vi "Read Images.vi"(8 "error in":errorcluster, 11 "Communicator Worker in":refnum<class "Camera Worker.lvclass">) -> (0 "error out":errorcluster, 3 "Communicator Worker out":refnum<class "Camera Worker.lvclass">)   [LabVIEW 2020, in "Camera Worker.lvlib" / "Camera Worker.lvclass"]
doc: "This method copies images from the camera's driver buffer into a local one."
uses:
  Camera Worker.lvclass
  Camera Worker.lvclass/Camera Worker.ctl
  Interfaces/IRead Image/IRead Images/IRead Image.lvclass
panel:
  out "Exec Time (ms)":u32
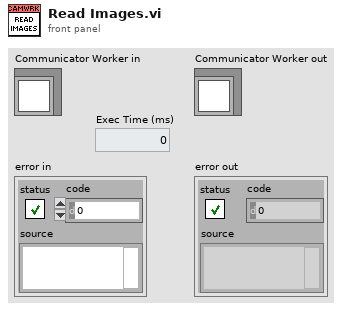
[diagram p1: front panel]
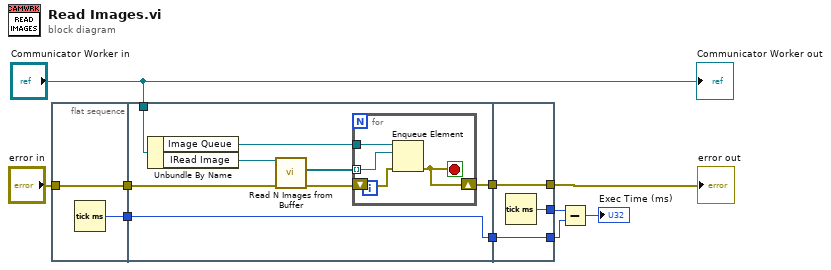
[diagram p0: block diagram]
diagram:
  n1 = flat-sequence {
    tunnel: "error in" -> [w12]
    tunnel: [w12] -> w7
    tunnel: [w11] -> w3
    tunnel: "Communicator Worker in" -> [w20]
    tunnel: w7 -> [w19]
    tunnel: [w16] -> w6
    tunnel: w3 -> [w13]
    tunnel: [w13] -> w2
    tunnel: [w27] -> w8
    tunnel: w6 -> [w27]
    tunnel: [w26] -> w5
    tunnel: [w25] -> w4
    tunnel: w2 -> [w25]
    frame #0 {
      n2 = Tick Count (ms)() -> (millisecond timer value=w11:u32)
    }
    frame #1 {
      n3 = Unbundle By Name(w20) -> ("Image Queue"=w18:refnum<queue>, "IRead Image"=w15:refnum<class "IRead Image.lvclass">)
      n4 = call-dynamic "Read N Images from Buffer.vi"("error in"=w19, "IRead Images in"=w15) -> ("error out"=w17:errorcluster, "images"=w14:refnum<class "Generic Image.lvclass">[])  [unwired: 7 in, 1 out]
      n5 = for {
        tunnel: w18 -> [w24]
        shift-right: [w21] -> w16
        shift-left: w17 -> [w23]
        tunnel: w14 -> [w22] mode=indexing
        stop <- w21 stop-if-true
        n6 = Enqueue Element(queue=w24, element=w22, error in (no error)=w23) -> (error out=w21:errorcluster)  [unwired: 1 in, 2 out]
      }
    }
    frame #2 {
      n7 = Tick Count (ms)() -> (millisecond timer value=w26:u32)
    }
  }
  n8 = Subtract(x=w5, y=w4) -> (x-y=→"Exec Time (ms)":u32)
  "error out" <- w8
  "Communicator Worker out" <- "Communicator Worker in"
